vi "Error Read.vi"(8 "error in":errorcluster, 11 "Error in":refnum<class "Error.lvclass">) -> (0 "error out":errorcluster, 1 "Changed or First Call?":bool, 2 "Error ACT":bool, 3 "Error out":refnum<class "Error.lvclass">)   [LabVIEW 2023, in "Error.lvclass"]
uses:
  Error.lvclass
  Error.lvclass/Error.ctl
  <vilib>/ADAS Replay HIL/Channels/Tag Wrapper/Polymorphic/Read Channel (Boolean).vi
  63493c8e-8c2e-4189-a001-8f899d062b19.vi
  <vilib>/ADAS Replay HIL/Channels/Tag Wrapper/Polymorphic/Read Channel (Boolean).vi/b2f764de-0c1e-4784-a155-687fc995a684.vi
  <vilib>/ADAS Replay HIL/Channels/Tag Wrapper/Polymorphic/Read Channel (Boolean).vi/b2f764de-0c1e-4784-a155-687fc995a684.vi/c28b0ead-42ad-4072-80a2-aca7f2bd7ce3.vi
  <vilib>/ADAS Replay HIL/Channels/Tag Wrapper/Polymorphic/Read Channel (Boolean).vi/b2f764de-0c1e-4784-a155-687fc995a684.vi/219d0231-d98b-4193-b5cc-84f90e3c9091.vi
  <vilib>/ADAS Replay HIL/Channels/Tag Wrapper/Tag Wrapper.lvlib
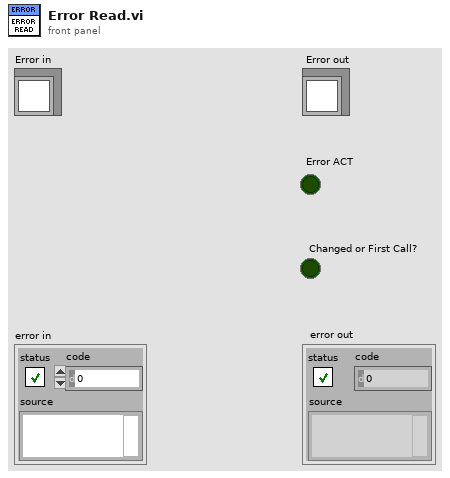
[diagram p1: front panel]
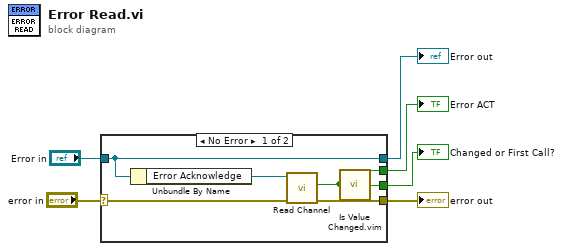
[diagram p0: block diagram]
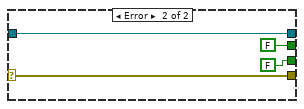
[diagram p2: hidden frame]
diagram:
  n1 = case shown="No Error" "error in" {
    selector: "error in" -> [w11 w16]
    tunnel: [w10 w16] -> w1
    tunnel: [w12 FALSE ("changed or first call?")] -> w3
    tunnel: "Error in" -> [w9 w13]
    tunnel: [w7 FALSE] -> w4
    tunnel: [w9 w13] -> w5
    frame No Error {
      n2 = Unbundle By Name(w9) -> ("Error Acknowledge"=w8:refnum<k21>)
      n3 = call-poly <vilib>:"Read Channel.vi"("error in"=w11, "ADAS HIL Channel in"=w8) -> ("error out"=w10:errorcluster, "Value out"=w7:bool)  [unwired: 6 in, 2 out]
      n4 = call "Is Value Changed.vim"("value"=w7) -> ("changed or first call?"=w12:bool)
    }
    frame Error {
    }
  }
  "Error out" <- w5
  "error out" <- w1
  "Changed or First Call?" <- w3
  "Error ACT" <- w4
